vi "PickPoint.vi"(8 "error in (no error)":errorcluster, 10 "Point":T2, 11 "SceneGraphDisplay in":refnum<class "SceneGraphDisplay.lvclass">) -> (0 "error out":errorcluster, 1 "Hit":bool, 2 "PickPoint":T1, 3 "SceneGraphDisplay out":refnum<class "SceneGraphDisplay.lvclass">)   [LabVIEW 2023, in "SceneGraphDisplay.lvclass"]
doc: "Given an x and y coordinate, casts a ray through the 3D scene and returns the x, y, and z-coordinates of the first object the ray intersects.\n\nQControl Class wrapper around the <b>SceneGraphDisplay : PickPoint Method</b>.\n<b> </b> <b> </b>\n©2016 Q Software Innovations, LLC (QSI)\nwritten by Quentin Alldredge\nproduced in LabVIEW 2015\n\nsupport@qsoftwareinnovations.com\nwww.qsoftwareinnovations.com\n\nAll rights reserved.\n\nRedistribution and use in source and binary forms, with or without modification, are permitted provided that the following conditions are met:\n\n * Redistributions of source code must retain the above copyright notice, this list of conditions and the following disclaimer.\n * Redistributions in binary form must reproduce the above copyright notice, this list of conditions and the following disclaimer in the documentation and/or other materials provided with the distribution.\n * Neither the name of Q Software Innovations, LLC. nor the names of its contributors may be used to endorse or promote products derived from this software without specific prior written permission.\n\nTHIS SOFTWARE IS PROVIDED BY THE COPYRIGHT HOLDERS AND CONTRIBUTORS \"AS IS\" AND ANY EXPRESS OR IMPLIED WARRANTIES, INCLUDING, BUT NOT LIMITED TO, THE IMPLIED WARRANTIES OF MERCHANTABILITY AND FITNESS FOR A PARTICULAR PURPOSE ARE DISCLAIMED. IN NO EVENT SHALL THE COPYRIGHT OWNER OR CONTRIBUTORS BE LIABLE FOR ANY DIRECT, INDIRECT, INCIDENTAL, SPECIAL, EXEMPLARY, OR CONSEQUENTIAL DAMAGES (INCLUDING, BUT NOT LIMITED TO, PROCUREMENT OF SUBSTITUTE GOODS OR SERVICES; LOSS OF USE, DATA, OR PROFITS; OR BUSINESS INTERRUPTION) HOWEVER CAUSED AND ON ANY THEORY OF LIABILITY, WHETHER IN CONTRACT, STRICT LIABILITY, OR TORT (INCLUDING NEGLIGENCE OR OTHERWISE) ARISING IN ANY WAY OUT OF THE USE OF THIS SOFTWARE, EVEN IF ADVISED OF THE POSSIBILITY OF SUCH DAMAGE."
uses:
  SceneGraphDisplay.lvclass
  <vilib>/Utility/miscctls.llb/LVPoint32TypeDef.ctl
  <vilib>/Utility/miscctls.llb/LV3DPointTypeDef.ctl
  SceneGraphDisplay.lvclass/SceneGraphDisplay.ctl
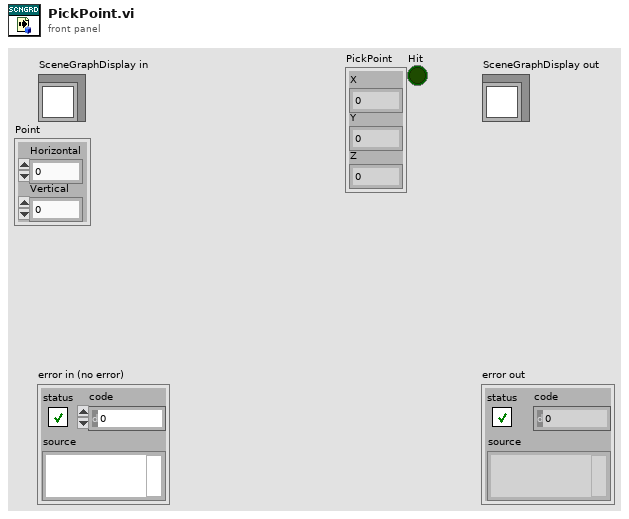
[diagram p1: front panel]
types:
  T1 = typedef "LV3DPointTypeDef.ctl" = cluster{"X":sgl, "Y":sgl, "Z":sgl}
  T2 = typedef "LVPoint32TypeDef.ctl" = cluster{"Horizontal":i32, "Vertical":i32}
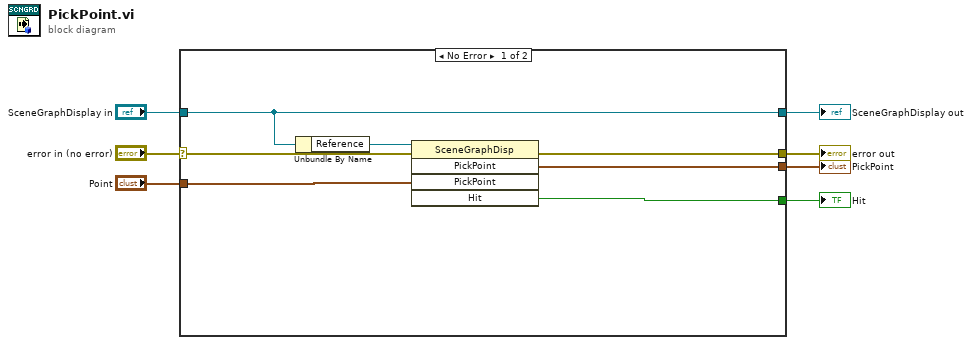
[diagram p0: block diagram]
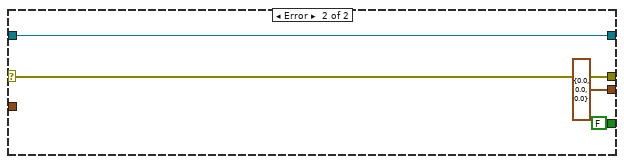
[diagram p2: hidden frame]
diagram:
  n1 = case shown="No Error" "error in (no error)" {
    selector: "error in (no error)" -> [w14 w18]
    tunnel: [w13 w18] -> w6
    tunnel: [w12 w17] -> w4
    tunnel: "SceneGraphDisplay in" -> [w12 w17]
    tunnel: "Point" -> [w10 _]
    tunnel: [w9 T1 {"X"=0.0, "Y"=0.0, "Z"=0.0} ("PickPoint")] -> w2
    tunnel: [w8 FALSE ("Hit")] -> w1
    frame No Error {
      n2 = Unbundle By Name(w12) -> ("Reference"=w11:refnum<vi>)
      n3 = invoke class="SceneGraphDisp" method="PickPoint"(reference=w11, error in=w14, "PickPoint"=w10) -> (error out=w13:errorcluster, "PickPoint"=w9:T1, "Hit"=w8:bool)  [unwired: 2 in, 2 out]
    }
    frame Error {
    }
  }
  "error out" <- w6
  "SceneGraphDisplay out" <- w4
  "PickPoint" <- w2
  "Hit" <- w1
